vi "Tester.vi"(8 "error in (no error)":errorcluster, 11 "Selector in":refnum<class "Selector.lvclass">) -> (0 "error out":errorcluster, 3 "Selector out":refnum<class "Selector.lvclass">)   [LabVIEW 2019, in "Selector.lvclass"]
uses:
  Selector.lvclass
  <vilib>/Utility/miscctls.llb/LVPositionTypeDef.ctl
panel:
  out "Events":string[](array[string])
  in  "Multicolumn Listbox":i32(listbox)
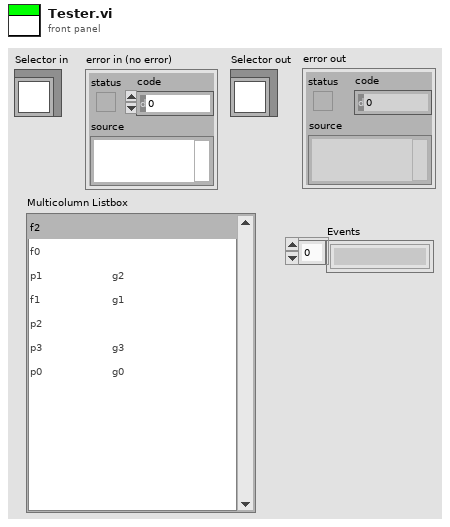
[diagram p1: front panel]
types:
  T1 = typedef "LVPositionTypeDef.ctl" = cluster{"Left":i32, "Top":i32}
  T2 = cluster{"Point":T1, "Button":u16, "PlatMods":cluster{"Shift":bool, "Ctrl":bool, "Alt":bool, "Cmd":bool, "Opt":bool}}
  T3 = enum32{"Invalid", "Standard", "Closed", "Hidden", "Minimized", "Maximized"}
  T4 = enum32{"invalid app kind", "Development System", "Run Time System", "Student Edition", "Embedded LabVIEW", "Evaluation", "Custom"}
  T5 = cluster{"Core":cluster{"Current VI Reference":refnum<vi>, "Close Panel on Exit?":bool}, "menu path":string}
  T6 = typedef "LVPoint32TypeDef.ctl" = cluster{"Horizontal":i32, "Vertical":i32}
  T7 = cluster{"Shift":bool, "Ctrl":bool, "Alt":bool, "Cmd":bool, "Opt":bool}
  T8 = cluster{"Current VI Reference":refnum<vi>, "Close Panel on Exit?":bool}
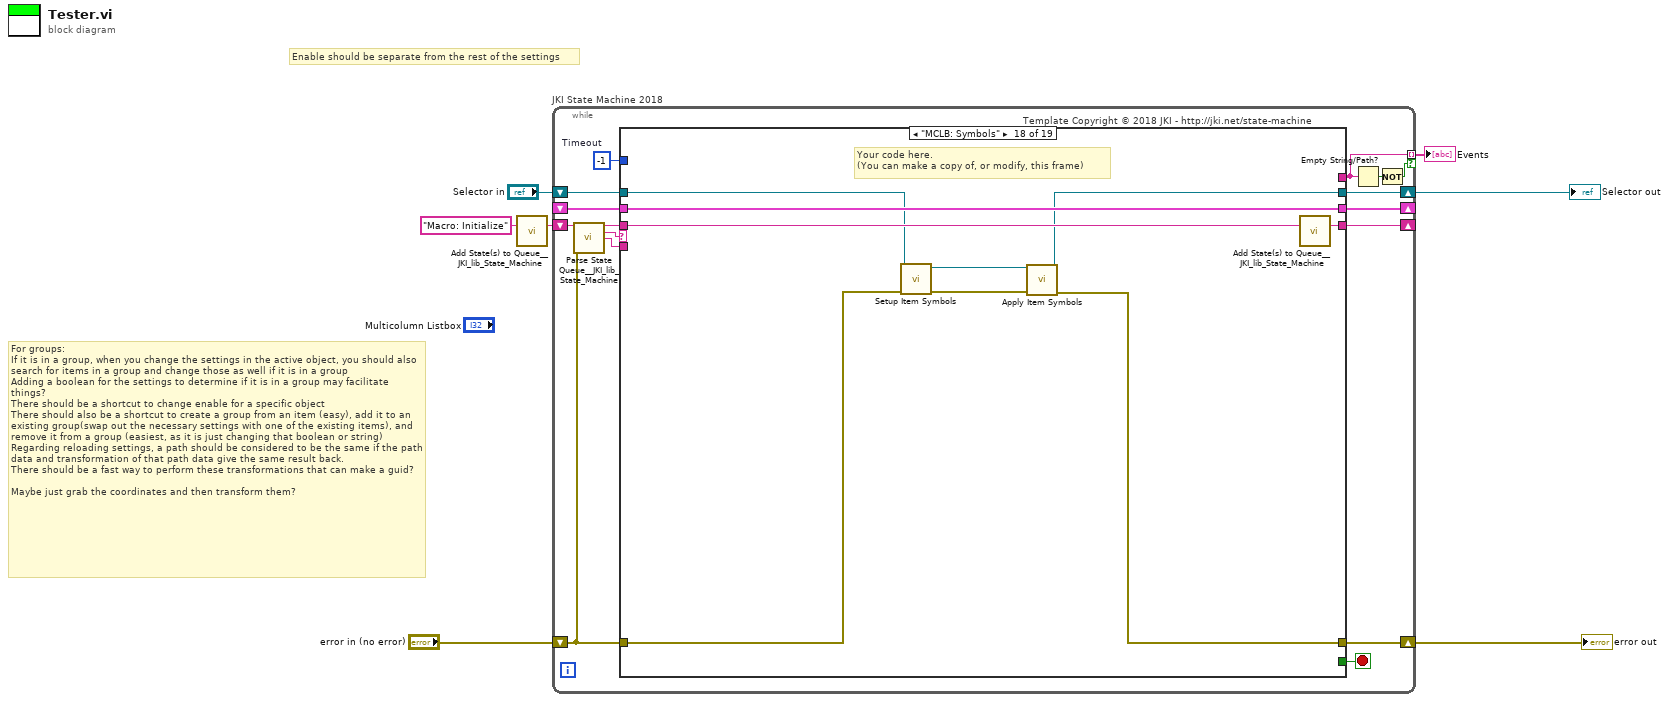
[diagram p0: block diagram]
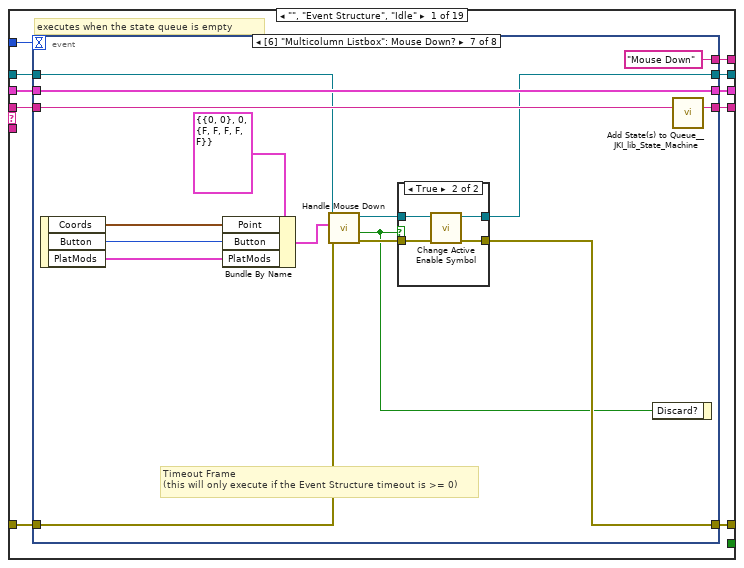
[diagram p2: hidden frame]
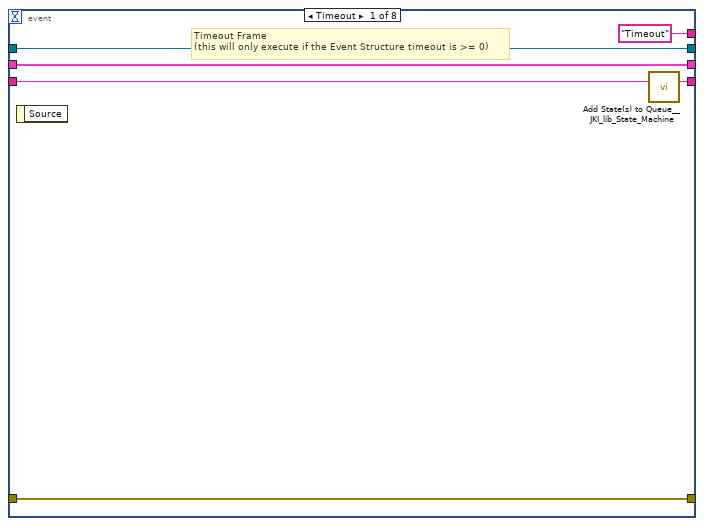
[diagram p3: hidden frame]
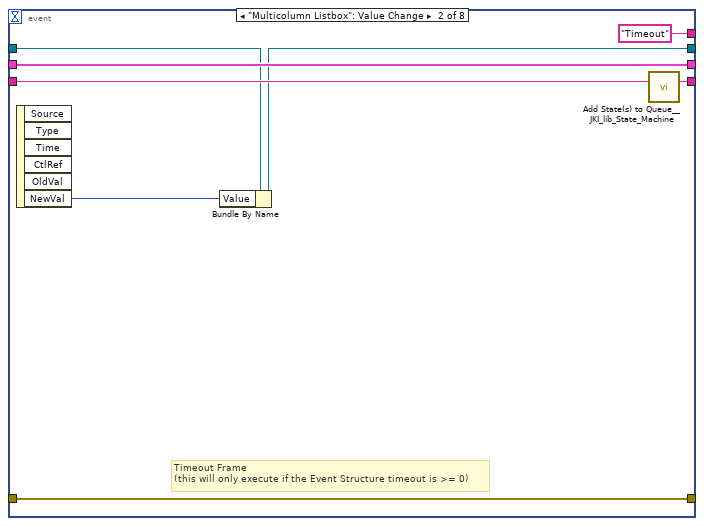
[diagram p4: hidden frame]
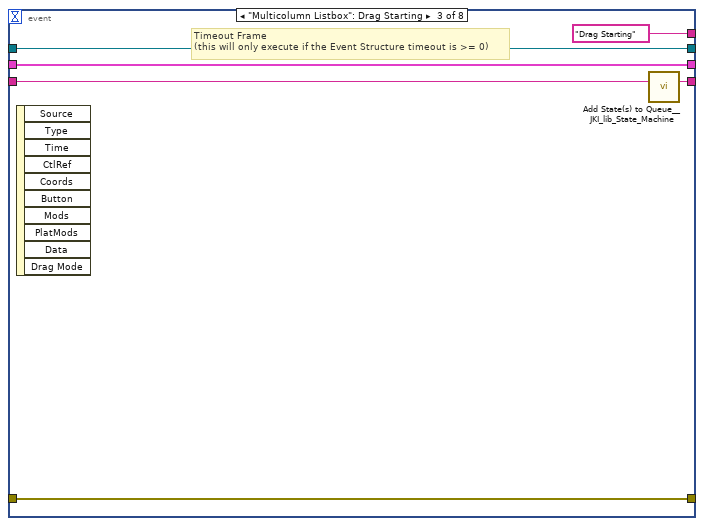
[diagram p5: hidden frame]
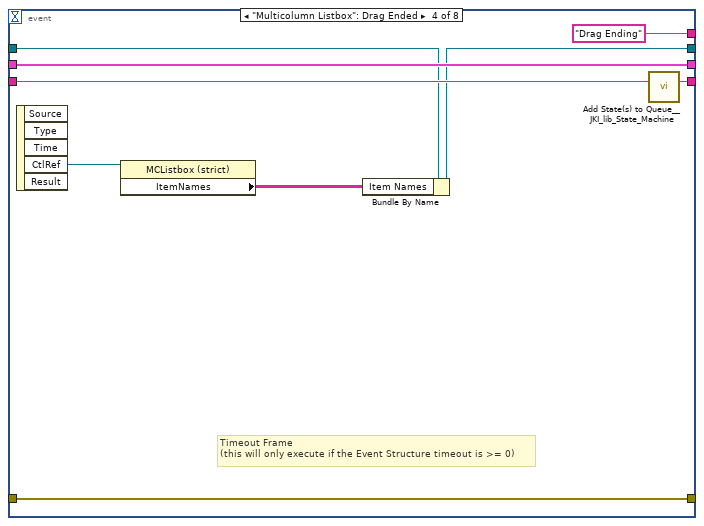
[diagram p6: hidden frame]
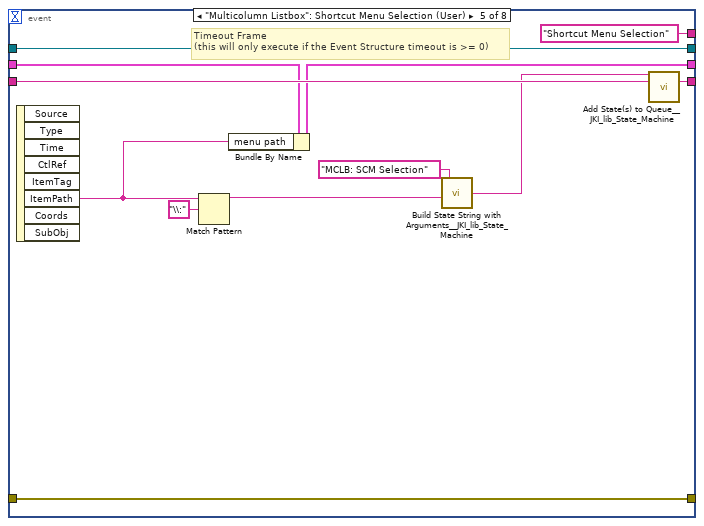
[diagram p7: hidden frame]
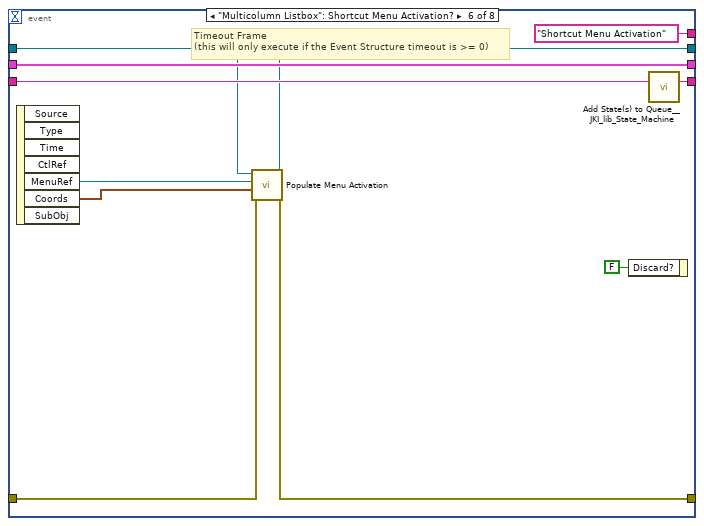
[diagram p8: hidden frame]
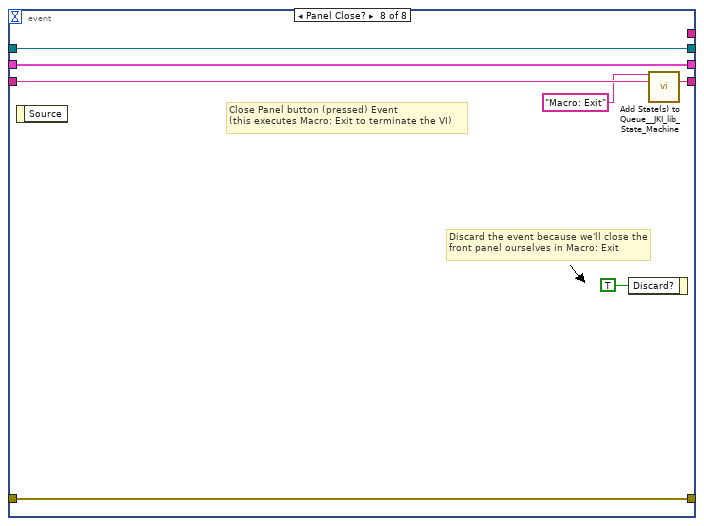
[diagram p10: hidden frame]
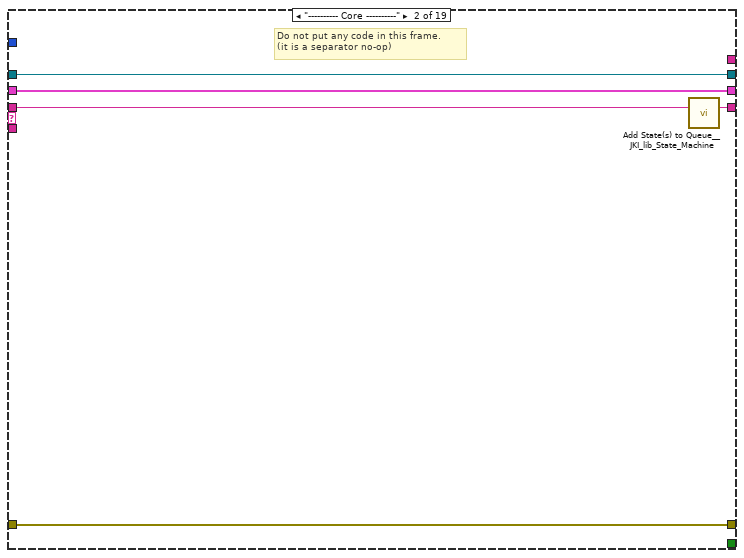
[diagram p11: hidden frame]
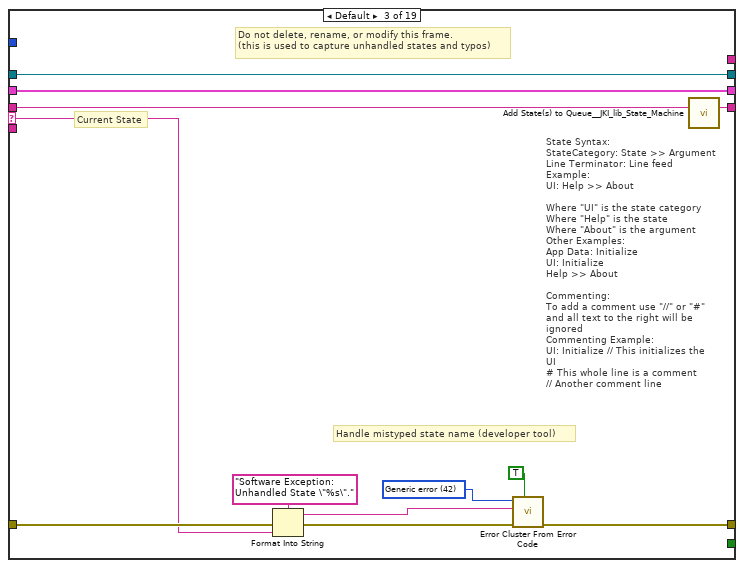
[diagram p12: hidden frame]
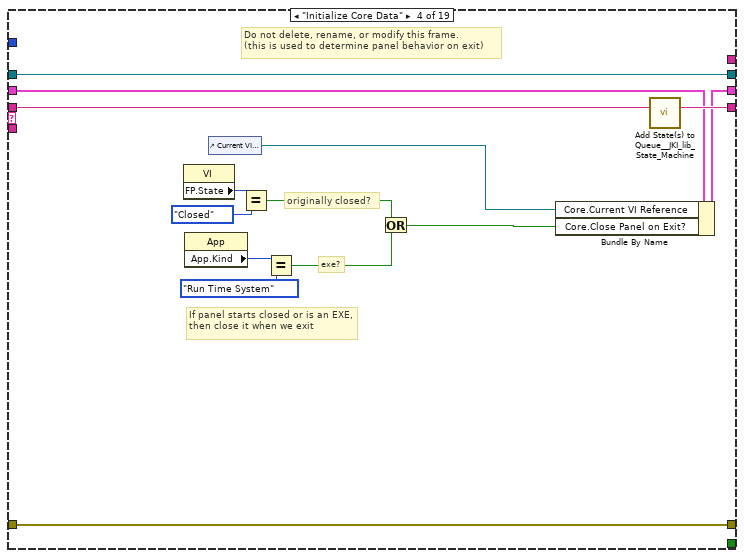
[diagram p13: hidden frame]
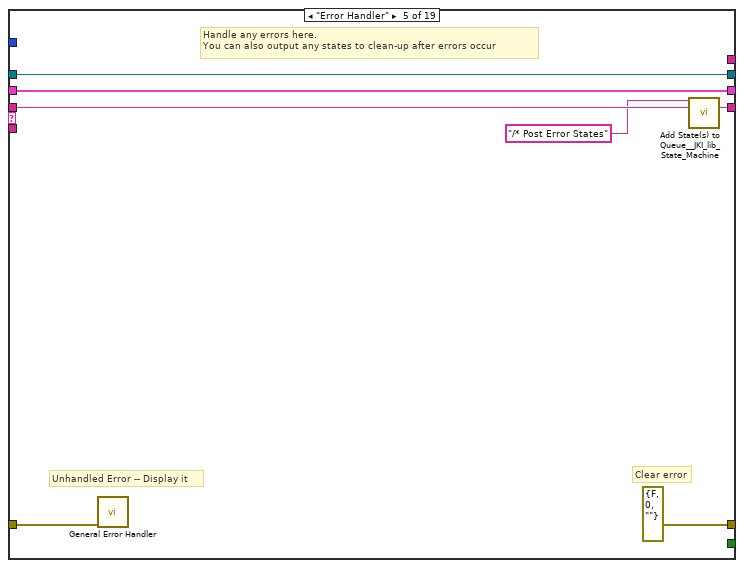
[diagram p14: hidden frame]
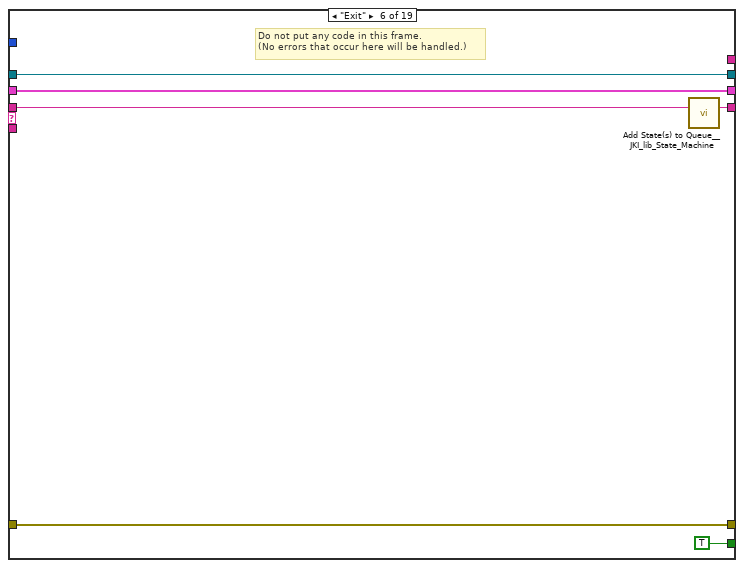
[diagram p15: hidden frame]
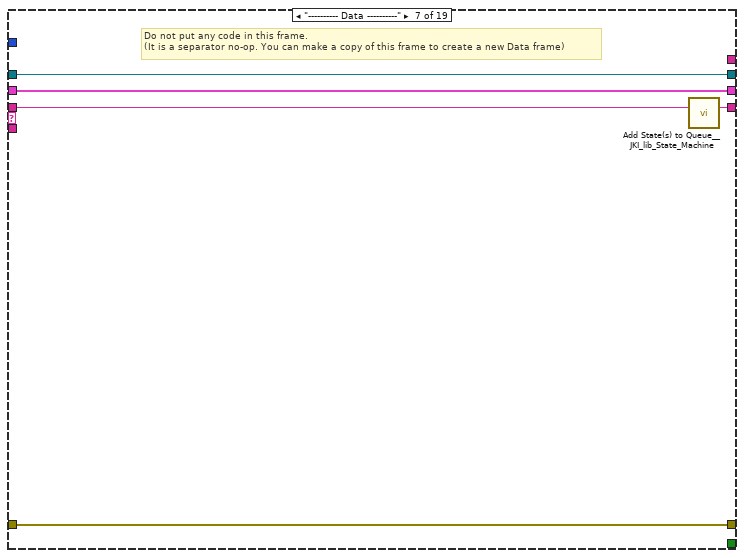
[diagram p16: hidden frame]
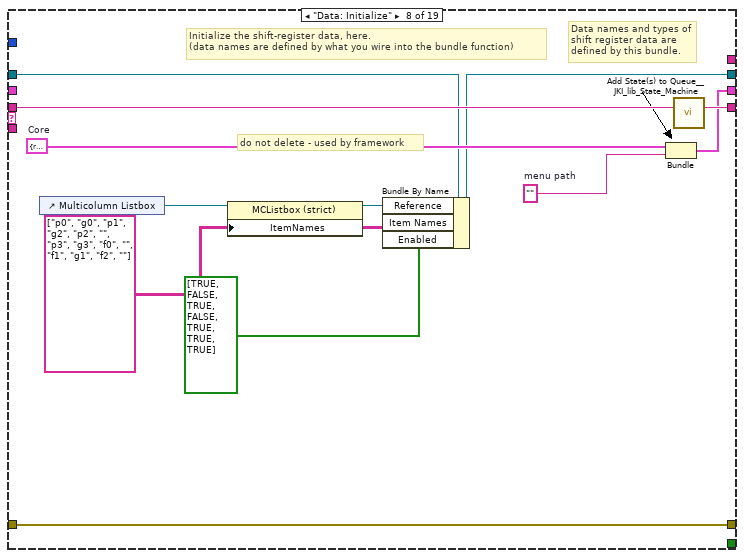
[diagram p17: hidden frame]
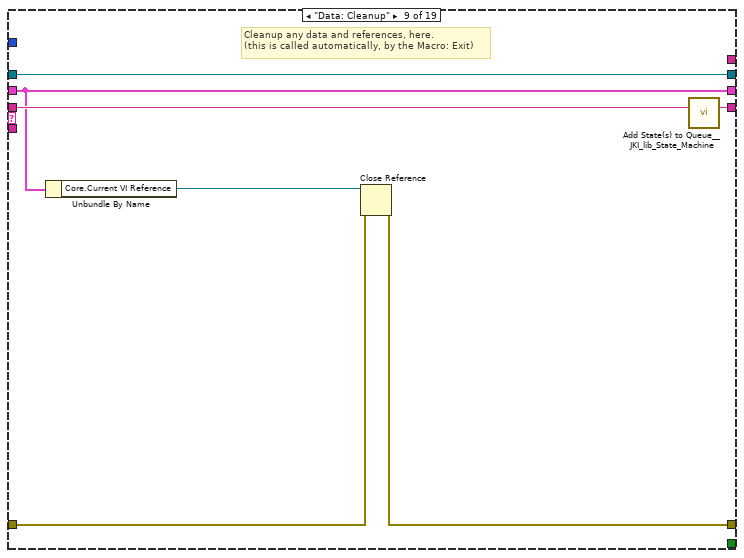
[diagram p18: hidden frame]
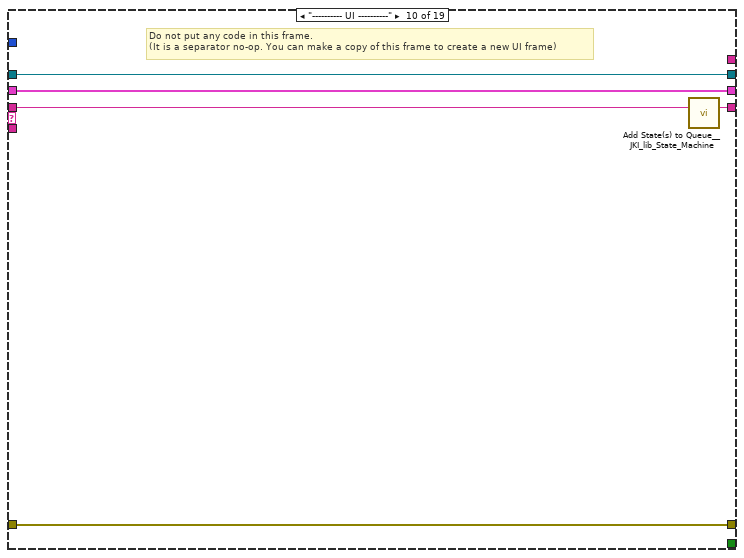
[diagram p19: hidden frame]
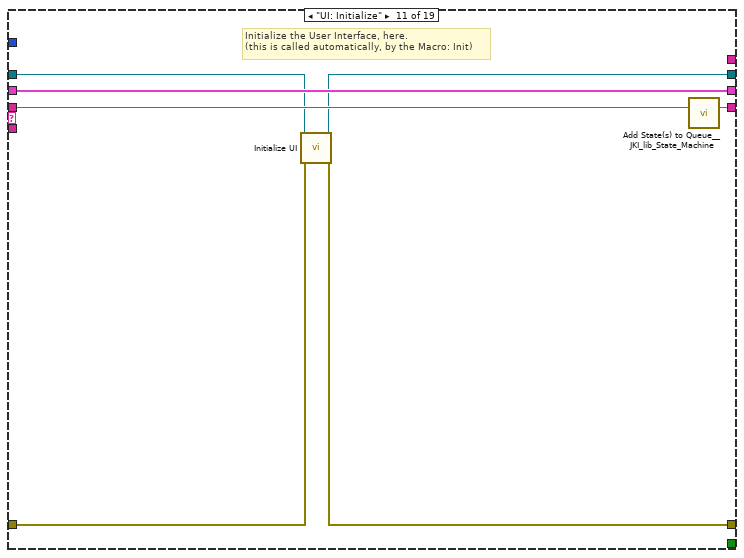
[diagram p20: hidden frame]
diagram:
  # "For groups:\nIf it is in a group, when you change the settings in the active object, you should also search for items in a group and change those as well if it is in a group \nAdding a boolean for the settings to determine if it is in a group may facilitate things?\nThere should be a shortcut to change enable for a specific object\nThere should also be a shortcut to create a group from an item (easy), add it to an existing group(swap out the necessary settings with one of the existing items), and remove it from a group (easiest, as it is just changing that boolean or string)\nRegarding reloading settings, a path should be considered to be the same if the path data and transformation of that path data give the same result back.\nThere should be a fast way to perform these transformations that can make a guid?\n\nMaybe just grab the coordinates and then transform them?"
  # "Enable should be separate from the rest of the settings"
  n1 = call <vilib>:"Add State(s) to Queue__JKI_lib_State_Machine.vi"("State(s) in (\"\")"="Macro: Initialize") -> ("States Out"=w7:string)  [unwired: 14 in]
  n2 = while "JKI State Machine 2018" {
    shift-right: [w16] -> _
    shift-left: _ -> [w15]
    shift-right: [w19] -> w2
    shift-left: "error in (no error)" -> [w13]
    shift-right: [w18] -> _
    shift-left: w7 -> [w20]
    shift-right: [w11] -> w4
    shift-left: "Selector in" -> [w12]
    tunnel: [w10] -> w1 mode=indexing if=w8
    stop <- w17 stop-if-true
    w14 = -1  # Timeout
    # "Template Copyright © 2018 JKI - http://jki.net/state-machine"
    n3 = call <vilib>:"Parse State Queue__JKI_lib_State_Machine.vi"("State Queue"=w20, "Error In (no error)"=w13) -> ("Remaining States"=w22:string, "Current State"=w23:string, "Arguments"=w21:string)  [unwired: 11 in]
    n4 = case shown="\"MCLB: Symbols\"" w23 {
      selector: w23 -> [_ _ w121 _ _ _ _ _ _ _ _ _ _ _ _ _ _ _ _]
      tunnel: w22 -> [w33 w119 w125 w145 w152 w158 w163 w175 w182 w187 w194 w201 w213 w283 w289 w300 w305 w314 w322]
      tunnel: w21 -> [_ _ _ _ _ _ _ _ _ _ _ w196 w207 _ _ _ _ _ w319]
      tunnel: w15 -> [w31 w116 w123 w138 w149 w156 w160 _ w177 w184 w192 w199 w209 w280 w286 w297 w302 w312 w316]
      tunnel: [w30 w117 w127 w142 errorcluster {"status"=FALSE, "code"=0, "source"=""} ("error out") w155 w161 w172 w178 w185 w189 w197 w210 w281 w287 w298 w303 w307 w320] -> w19
      tunnel: w13 -> [w29 w117 w126 w142 w148 w155 w161 w172 w179 w185 w188 w198 w211 w281 w287 w298 w303 w306 w320]
      tunnel: [w32 w118 w124 w144 w151 w157 w162 w174 w181 w186 w193 w200 w212 w282 w288 w299 w304 w313 w321] -> w18
      tunnel: [_ _ _ _ _ TRUE _ _ _ _ _ _ _ _ _ _ _ _ _] -> w17
      tunnel: [w28 w116 w123 w143 w149 w156 w160 w173 w177 w184 w192 w199 w209 w280 w286 w297 w302 w312 w316] -> w16
      tunnel: w14 -> [w27 _ _ _ _ _ _ _ _ _ _ _ _ _ _ _ _ _ _]
      tunnel: w12 -> [w26 w115 w120 w132 w146 w153 w159 w169 w176 w183 w190 w195 w206 w279 w284 w290 w301 w311 w317]
      tunnel: [w25 w115 w120 w132 w146 w153 w159 w170 w176 w183 w191 w195 w206 w279 w284 w290 w301 w308 w318] -> w11
      tunnel: [w24 _ _ _ _ _ _ _ _ _ _ _ _ _ _ _ _ _ _] -> w10
      frame "", "Event Structure", "Idle" {
        # "executes when the state queue is empty"
        n5 = event shown="[6] \"Multicolumn Listbox\": Mouse Down?" {
          selector: _ -> [_ _ _ _ _ _ _ _]
          dyn-events: _ -> [_ _ _ _ _ _ _ _]
          timeout: w27 -> [_ _ _ _ _ _ _ _]
          tunnel: w33 -> [w39 w47 w53 w62 w74 w85 w101 w114]
          tunnel: [w38 w46 w52 w61 w73 w84 w100 w113] -> w32
          tunnel: w31 -> [w36 w44 w50 w59 w67 w83 w99 w111]
          tunnel: [w37 w45 w51 w60 w72 w78 w91 w112] -> w30
          tunnel: w29 -> [w37 w45 w51 w60 w72 w77 w97 w112]
          tunnel: [w36 w44 w50 w59 w68 w83 w99 w111] -> w28
          tunnel: w26 -> [w35 w41 w49 w55 w71 w76 w98 w108]
          tunnel: [w35 w42 w49 w56 w71 w82 w89 w108] -> w25
          tunnel: ["Timeout" "Timeout" "Drag Starting" "Drag Ending" "Shortcut Menu Selection" "Shortcut Menu Activation" "Mouse Down" _] -> w24
          event Timeout {
            # "Timeout Frame\n(this will only execute if the Event Structure timeout is >= 0)"
            n6 = event-data() -> ()  [unwired: 1 in, 1 out]
            n7 = call <vilib>:"Add State(s) to Queue__JKI_lib_State_Machine.vi"("State(s) in (\"\")"=w39) -> ("States Out"=w38:string)  [unwired: 14 in]
          }
          event "Multicolumn Listbox": Value Change {
            # "Timeout Frame\n(this will only execute if the Event Structure timeout is >= 0)"
            n8 = event-data() -> ("NewVal"=w40:i32)  [unwired: 1 in, 5 out]
            n9 = Bundle By Name(cluster=w41, "Value"=w40) -> (w42:refnum<class "Selector.lvclass">)
            n10 = call <vilib>:"Add State(s) to Queue__JKI_lib_State_Machine.vi"("State(s) in (\"\")"=w47) -> ("States Out"=w46:string)  [unwired: 14 in]
          }
          event "Multicolumn Listbox": Drag Starting {
            # "Timeout Frame\n(this will only execute if the Event Structure timeout is >= 0)"
            n11 = event-data() -> ()  [unwired: 1 in, 10 out]
            n12 = call <vilib>:"Add State(s) to Queue__JKI_lib_State_Machine.vi"("State(s) in (\"\")"=w53) -> ("States Out"=w52:string)  [unwired: 14 in]
          }
          event "Multicolumn Listbox": Drag Ended {
            # "Timeout Frame\n(this will only execute if the Event Structure timeout is >= 0)"
            n13 = event-data() -> ("CtlRef"=w57:refnum<vi>)  [unwired: 1 in, 4 out]
            n14 = property class="MCListbox (strict)"(reference=w57) -> ("ItemNames"=w54:string[][])  [unwired: 1 in, 2 out]
            n15 = Bundle By Name(cluster=w55, "Item Names"=w54) -> (w56:refnum<class "Selector.lvclass">)
            n16 = call <vilib>:"Add State(s) to Queue__JKI_lib_State_Machine.vi"("State(s) in (\"\")"=w62) -> ("States Out"=w61:string)  [unwired: 14 in]
          }
          event "Multicolumn Listbox": Shortcut Menu Selection (User) {
            # "Timeout Frame\n(this will only execute if the Event Structure timeout is >= 0)"
            n17 = event-data() -> ("ItemPath"=w69:string)  [unwired: 1 in, 7 out]
            n18 = Match Pattern(string=w69, regular expression="\\:") -> (before substring=w65:string)  [unwired: 1 in, 3 out]
            n19 = Bundle By Name(cluster=w67, "menu path"=w69) -> (w68:T5)
            n20 = call <vilib>:"Build State String with Arguments__JKI_lib_State_Machine.vi"("Arguments (\"\")"=w65, "State"="MCLB: SCM Selection") -> ("State with Arguments"=w64:string)  [unwired: 4 in]
            n21 = call <vilib>:"Add State(s) to Queue__JKI_lib_State_Machine.vi"("State(s) in Front (\"\")"=w64, "State(s) in (\"\")"=w74) -> ("States Out"=w73:string)  [unwired: 13 in]
          }
          event "Multicolumn Listbox": Shortcut Menu Activation? {
            # "Timeout Frame\n(this will only execute if the Event Structure timeout is >= 0)"
            n22 = event-data() -> ("MenuRef"=w81:refnum<k9>, "Coords"=w80:T6)  [unwired: 1 in, 5 out]
            n23 = call-dynamic "Populate Menu Activation.vi"("error in (no error)"=w77, "Point32"=w80, "MenuRef"=w81, "Selector in"=w76) -> ("error out"=w78:errorcluster, "Selector out"=w82:refnum<class "Selector.lvclass">)  [unwired: 6 in]
            n24 = event-data("Discard?"=FALSE) -> ()  [unwired: 1 in, 1 out]
            n25 = call <vilib>:"Add State(s) to Queue__JKI_lib_State_Machine.vi"("State(s) in (\"\")"=w85) -> ("States Out"=w84:string)  [unwired: 14 in]
          }
          event "Multicolumn Listbox": Mouse Down? {
            # "Timeout Frame\n(this will only execute if the Event Structure timeout is >= 0)"
            n26 = event-data() -> ("Coords"=w94:T6, "Button"=w93:u16, "PlatMods"=w95:T7)  [unwired: 1 in]
            n27 = Bundle By Name(cluster=T2 {"Point"={"Left"=0, "Top"=0}, "Button"=0, "PlatMods"={"Shift"=FALSE, "Ctrl"=FALSE, "Alt"=FALSE, "Cmd"=FALSE, "Opt"=FALSE}} ("Event Data"), "Point"=w94, "Button"=w93, "PlatMods"=w95) -> (w86:T2)
            n28 = call-dynamic "Handle Mouse Down.vi"("error in (no error)"=w97, "Event Data"=w86, "Selector in"=w98) -> ("error out"=w92:errorcluster, "Enable Change"=w87:bool, "Selector out"=w90:refnum<class "Selector.lvclass">)  [unwired: 6 in]
            n29 = case shown="True" w87 {
              tunnel: w90 -> [w103 w107]
              tunnel: w92 -> [w102 w106]
              tunnel: [w102 w105] -> w91
              tunnel: [w103 w104] -> w89
              frame False {
              }
              frame True {
                n30 = call "Change Active Enable Symbol.vi"("error in (no error)"=w106, "Selector in"=w107) -> ("error out"=w105:errorcluster, "Selector out"=w104:refnum<class "Selector.lvclass">)  [unwired: 8 in]
              }
            }
            n31 = event-data("Discard?"=w87) -> ()  [unwired: 1 in, 1 out]
            n32 = call <vilib>:"Add State(s) to Queue__JKI_lib_State_Machine.vi"("State(s) in (\"\")"=w101) -> ("States Out"=w100:string)  [unwired: 14 in]
          }
          event Panel Close? {
            # "Discard the event because we'll close the front panel ourselves in Macro: Exit"
            # "Close Panel button (pressed) Event\n(this executes Macro: Exit to terminate the VI)"
            n33 = event-data() -> ()  [unwired: 1 in, 1 out]
            n34 = event-data("Discard?"=TRUE) -> ()  [unwired: 1 in, 1 out]
            n35 = call <vilib>:"Add State(s) to Queue__JKI_lib_State_Machine.vi"("State(s) in Front (\"\")"="Macro: Exit", "State(s) in (\"\")"=w114) -> ("States Out"=w113:string)  [unwired: 13 in]
          }
        }
      }
      frame "---------- Core ----------" {
        # "Do not put any code in this frame.\n(it is a separator no-op)"
        n36 = call <vilib>:"Add State(s) to Queue__JKI_lib_State_Machine.vi"("State(s) in (\"\")"=w119) -> ("States Out"=w118:string)  [unwired: 14 in]
      }
      frame Default {
        w130 = 42 items=["No error", "Argument error", "Memory is full", "Out of zone", "End of file", "File already open", "Generic file I/O error", "File not found", "File permission error", "Disk is full", "Duplicate path", "Too many files open", "System feature not enabled", "Resource file not found", "Cannot add resource", "Resource not found", "Image not found", "Image memory error", "Pen does not exist", "Config type invalid", "Config token not found", "Config parse error", "Config memory error", "Bad external code format", "Bad external code offset", "External code not present", "Null window", "Destroy window error", "Null menu", "Print aborted", "Bad print record", "Print driver error", "Windows error during printing", "Memory error during printing", "Print dialog error", "Generic print error", "Invalid device refnum", "Device not found", "Device parameter error", "Device unit error", "Cannot open device", "Device call aborted", "Generic error", "Cancelled by user", "Object ID too low", "Object ID too high", "Object not in heap", "Unknown heap", "Unknown object (invalid DefProc)", "Unknown object (DefProc not in table)", "Message out of range", "Invalid (null) method", "Unknown message", "Manager call not supported", "Bad address", "Network operation in progress", "Network operation timed out", "Connection is busy", "Network attribute not supported", "Network error", "Address in use", "System out of memory", "Connection aborted", "Connection refused", "Not connected", "Already connected", "Connection closed", "Initialization error (interapplication manager)", "Bad occurrence", "Wait on unbound occurrence handler", "Occurrence queue overflow", "Datalog type conflict", "Unused", "Unrecognized type (interapplication manager)", "Memory corrupt", "Failed to make temporary DLL", "Old CIN version", "Drag socket not found", "Failed to load drop-object", "Failed to register OLE object", "Failed to release OLE object", "Format specifier type mismatch", "Unknown format specifier", "Too few format specifiers", "Too many format specifiers", "Scan failed", "Newer CIN version", "Error converting to variant", "Runtime menu error", "Password tampered", "Variant attribute not found", "Incompatible variant data type", "Event data is not available", "Event Store is not present", "Occurrence is not found", "Event Queue is not created", "Event info is not available", "Refnum passed is NULL", "Error retrieving Class GUID", "Error retrieving CoClass GUID", "Error retrieving TypeLib GUID.", "Bad built application magic bytes.", "Specific driver is different from the specific driver associated with the Logical Name.", "There is no session opened to the class driver.", "Max Error", "MAX - Error with config objects", "MAX - Error loading configuration", "MAX - Group not supported"]
        # "State Syntax:\nStateCategory: State >> Argument\nLine Terminator: Line feed\nExample:\nUI: Help >> About\n\nWhere \"UI\" is the state category\nWhere \"Help\" is the state\nWhere \"About\" is the argument\nOther Examples:\nApp Data: Initialize\nUI: Initialize\nHelp >> About\n\nCommenting:\nTo add a comment use \"//\" or \"#\" and all text to the right will be ignored\nCommenting Example:\nUI: Initialize // This initializes the UI\n# This whole line is a comment\n// Another comment line"
        # "Current State"
        # "Do not delete, rename, or modify this frame.\n(this is used to capture unhandled states and typos)"
        # "Handle mistyped state name (developer tool)"
        n37 = Format Into String(format string="Software Exception: Unhandled State \"%s\"." ("message"), error in=w126, w121) -> (resulting string=w129:string, error out=w128:errorcluster)  [unwired: 1 in]
        n38 = call <vilib>:"Error Cluster From Error Code.vi"("show call chain? (False)"=TRUE, "error in (no error)"=w128, "error message (\"\")"=w129, "error code (0)"=w130) -> ("error out"=w127:errorcluster)  [unwired: 5 in]
        n39 = call <vilib>:"Add State(s) to Queue__JKI_lib_State_Machine.vi"("State(s) in (\"\")"=w125) -> ("States Out"=w124:string)  [unwired: 14 in]
      }
      frame "Initialize Core Data" {
        # "Do not delete, rename, or modify this frame.\n(this is used to determine panel behavior on exit)"
        # "originally closed?"
        # "exe?"
        # "If panel starts closed or is an EXE, then close it when we exit"
        n40 = property class="VI"() -> ("FP.State"=w135:T3)  [unwired: 2 in, 2 out]
        n41 = property class="App"() -> ("App.Kind"=w141:T4)  [unwired: 2 in, 2 out]
        n42 = control-ref of="Current VI Reference"() -> (w136:refnum<vi>)
        n43 = Equal?(x=w135, y=T3."Closed" ("Front Panel Window:State")) -> (x = y?=w133:bool)
        n44 = Equal?(x=w141, y=T4."Run Time System" ("Application:Kind")) -> (x = y?=w139:bool)
        n45 = Or(x=w133, y=w139) -> (x .or. y?=w137:bool)
        n46 = Bundle By Name(cluster=w138, "Core.Current VI Reference"=w136, "Core.Close Panel on Exit?"=w137) -> (w143:T5)
        n47 = call <vilib>:"Add State(s) to Queue__JKI_lib_State_Machine.vi"("State(s) in (\"\")"=w145) -> ("States Out"=w144:string)  [unwired: 14 in]
      }
      frame "Error Handler" {
        # "Unhandled Error -- Display it"
        # "Handle any errors here.\nYou can also output any states to clean-up after errors occur"
        # "Clear error"
        n48 = call <vilib>:"General Error Handler.vi"("error in (no error)"=w148) -> ()  [unwired: 10 in, 5 out]
        n49 = call <vilib>:"Add State(s) to Queue__JKI_lib_State_Machine.vi"("State(s) in Front (\"\")"="/* Post Error States", "State(s) in (\"\")"=w152) -> ("States Out"=w151:string)  [unwired: 13 in]
      }
      frame "Exit" {
        # "Do not put any code in this frame.\n(No errors that occur here will be handled.)"
        n50 = call <vilib>:"Add State(s) to Queue__JKI_lib_State_Machine.vi"("State(s) in (\"\")"=w158) -> ("States Out"=w157:string)  [unwired: 14 in]
      }
      frame "---------- Data ----------" {
        # "Do not put any code in this frame.\n(It is a separator no-op. You can make a copy of this frame to create a new Data frame)"
        n51 = call <vilib>:"Add State(s) to Queue__JKI_lib_State_Machine.vi"("State(s) in (\"\")"=w163) -> ("States Out"=w162:string)  [unwired: 14 in]
      }
      frame "Data: Initialize" {
        w164 = ""  # menu path
        w166 = string[][] [["p0", "g0"], ["p1", "g2"], ["p2", ""], ["p3", "g3"], ["f0", ""], ["f1", "g1"], ["f2", ""]] ("Item Names")
        w171 = T8 {"Current VI Reference"=refnum, "Close Panel on Exit?"=FALSE}  # Core
        # "do not delete - used by framework"
        # "Data names and types of shift register data are defined by this bundle."
        # "Initialize the shift-register data, here.\n(data names are defined by what you wire into the bundle function)"
        n52 = control-ref of="Multicolumn Listbox"() -> (w168:refnum<vi>)
        n53 = property class="MCListbox (strict)"(reference=w168, "ItemNames"=w166) -> (reference out=w167:refnum<vi>)  [unwired: 1 in, 1 out]
        n54 = Bundle By Name(cluster=w169, "Reference"=w167, "Item Names"=w166, "Enabled"=bool[] [TRUE, FALSE, TRUE, FALSE, TRUE, TRUE, TRUE]) -> (w170:refnum<class "Selector.lvclass">)
        n55 = Bundle("Core"=w171, "menu path"=w164) -> (w173:T5)  [unwired: 1 in]
        n56 = call <vilib>:"Add State(s) to Queue__JKI_lib_State_Machine.vi"("State(s) in (\"\")"=w175) -> ("States Out"=w174:string)  [unwired: 14 in]
      }
      frame "Data: Cleanup" {
        # "Cleanup any data and references, here.\n(this is called automatically, by the Macro: Exit)"
        n57 = Unbundle By Name(w177) -> ("Core.Current VI Reference"=w180:refnum<vi>)
        n58 = Close Reference(reference=w180, error in (no error)=w179) -> (error out=w178:errorcluster)
        n59 = call <vilib>:"Add State(s) to Queue__JKI_lib_State_Machine.vi"("State(s) in (\"\")"=w182) -> ("States Out"=w181:string)  [unwired: 14 in]
      }
      frame "---------- UI ----------" {
        # "Do not put any code in this frame.\n(It is a separator no-op. You can make a copy of this frame to create a new UI frame)"
        n60 = call <vilib>:"Add State(s) to Queue__JKI_lib_State_Machine.vi"("State(s) in (\"\")"=w187) -> ("States Out"=w186:string)  [unwired: 14 in]
      }
      frame "UI: Initialize" {
        # "Initialize the User Interface, here.\n(this is called automatically, by the Macro: Init)"
        n61 = call-dynamic "Initialize UI.vi"("error in (no error)"=w188, "Selector in"=w190) -> ("error out"=w189:errorcluster, "Selector out"=w191:refnum<class "Selector.lvclass">)  [unwired: 8 in]
        n62 = call <vilib>:"Add State(s) to Queue__JKI_lib_State_Machine.vi"("State(s) in (\"\")"=w194) -> ("States Out"=w193:string)  [unwired: 14 in]
      }
      frame "UI: Cursor Set" {
        # "Argument"
        # "Set and Unset Cursor Busy.\n(Usage: \"UI: Cursor Set >> Busy|Idle\")"
        n63 = case shown="\"Idle\", Default" w196 {
          tunnel: w198 -> [w203 w205]
          tunnel: [w202 w204] -> w197
          frame "Idle", Default {
            n64 = call <vilib>:"Unset Busy.vi"("error in (no error)"=w203) -> ("error out"=w202:errorcluster)  [unwired: 10 in]
          }
          frame "Busy" {
            n65 = call <vilib>:"Set Busy.vi"("error in (no error)"=w205) -> ("error out"=w204:errorcluster)  [unwired: 9 in, 1 out]
          }
        }
        n66 = call <vilib>:"Add State(s) to Queue__JKI_lib_State_Machine.vi"("State(s) in (\"\")"=w201) -> ("States Out"=w200:string)  [unwired: 14 in]
      }
      frame "UI: Front Panel State" {
        # "Argument"
        # "Set Front Panel Open or Closed\n(Usage: \"UI: Front Panel State >> Open|Close\")"
        n67 = Unbundle By Name(w209) -> ("Core.Current VI Reference"=w208:refnum<vi>)
        n68 = case shown="\"Minimize\", \"Minimized\"" w207 {
          tunnel: w211 -> [w219 w234 w245 w258 w271]
          tunnel: [w221 w235 w247 w260 w273] -> w210
          tunnel: w208 -> [w220 w232 w246 w259 w272]
          frame "Open", "Standard", Default {
            w214 = T3."Standard" ("State")
            n69 = property class="VI"(reference=w220, error in=w219) -> (reference out=w217:refnum<vi>, error out=w218:errorcluster, "FP.State"=w216:T3)
            n70 = Not Equal?(x=w216, y=w214) -> (x != y?=w215:bool)
            n71 = case shown="True" w215 {
              tunnel: [w225 w227] -> w221
              tunnel: w218 -> [w224 w227]
              tunnel: w217 -> [w223 _]
              tunnel: w214 -> [w222 _]
              frame True {
                n72 = invoke class="VI" method="FP.Open"(reference=w223, error in=w224, "Activate"=TRUE, "State"=w222) -> (error out=w225:errorcluster)  [unwired: 1 in, 4 out]
              }
              frame False {
              }
            }
          }
          frame "Close", "Closed" {
            n73 = property class="VI"(reference=w232, error in=w234) -> (reference out=w231:refnum<vi>, error out=w233:errorcluster, "FP.State"=w229:T3)
            n74 = Not Equal?(x=w229, y=T3."Closed" ("Front Panel Window:State")) -> (x != y?=w228:bool)
            n75 = case shown="True" w228 {
              tunnel: [w236 w239] -> w235
              tunnel: w233 -> [w236 w238]
              tunnel: w231 -> [_ w237]
              frame False {
              }
              frame True {
                n76 = invoke class="VI" method="FP.Close"(reference=w237, error in=w238) -> (error out=w239:errorcluster)  [unwired: 1 in, 2 out]
              }
            }
          }
          frame "Hidden", "Hide" {
            w240 = T3."Hidden" ("State")
            n77 = property class="VI"(reference=w246, error in=w245) -> (reference out=w243:refnum<vi>, error out=w244:errorcluster, "FP.State"=w242:T3)
            n78 = Not Equal?(x=w242, y=w240) -> (x != y?=w241:bool)
            n79 = case shown="True" w241 {
              tunnel: [w251 w252] -> w247
              tunnel: w244 -> [w250 w252]
              tunnel: w243 -> [w249 _]
              tunnel: w240 -> [w248 _]
              frame True {
                n80 = invoke class="VI" method="FP.Open"(reference=w249, error in=w250, "State"=w248) -> (error out=w251:errorcluster)  [unwired: 2 in, 4 out]
              }
              frame False {
              }
            }
          }
          frame "Minimize", "Minimized" {
            w253 = T3."Minimized" ("State")
            n81 = property class="VI"(reference=w259, error in=w258) -> (reference out=w256:refnum<vi>, error out=w257:errorcluster, "FP.State"=w255:T3)
            n82 = Not Equal?(x=w255, y=w253) -> (x != y?=w254:bool)
            n83 = case shown="True" w254 {
              tunnel: [w264 w265] -> w260
              tunnel: w257 -> [w263 w265]
              tunnel: w256 -> [w262 _]
              tunnel: w253 -> [w261 _]
              frame True {
                n84 = invoke class="VI" method="FP.Open"(reference=w262, error in=w263, "State"=w261) -> (error out=w264:errorcluster)  [unwired: 2 in, 4 out]
              }
              frame False {
              }
            }
          }
          frame "Maximize", "Maximized" {
            w266 = T3."Maximized" ("State")
            n85 = property class="VI"(reference=w272, error in=w271) -> (reference out=w269:refnum<vi>, error out=w270:errorcluster, "FP.State"=w268:T3)
            n86 = Not Equal?(x=w268, y=w266) -> (x != y?=w267:bool)
            n87 = case shown="True" w267 {
              tunnel: [w277 w278] -> w273
              tunnel: w270 -> [w276 w278]
              tunnel: w269 -> [w275 _]
              tunnel: w266 -> [w274 _]
              frame True {
                n88 = invoke class="VI" method="FP.Open"(reference=w275, error in=w276, "State"=w274) -> (error out=w277:errorcluster)  [unwired: 2 in, 4 out]
              }
              frame False {
              }
            }
          }
        }
        n89 = call <vilib>:"Add State(s) to Queue__JKI_lib_State_Machine.vi"("State(s) in (\"\")"=w213) -> ("States Out"=w212:string)  [unwired: 14 in]
      }
      frame "---------- Macro ----------" {
        # "Do not put any code in this frame.\n(It is a separator no-op. You can make a copy of this frame to create a new Macro frame)"
        n90 = call <vilib>:"Add State(s) to Queue__JKI_lib_State_Machine.vi"("State(s) in (\"\")"=w283) -> ("States Out"=w282:string)  [unwired: 14 in]
      }
      frame "Macro: Initialize" {
        # "Initialization Macro\n(This is called once, when the VI starts)"
        n91 = call <vilib>:"Add State(s) to Queue__JKI_lib_State_Machine.vi"("State(s) in Front (\"\")"="Data: Initialize\nInitialize Core Data\nUI: Initialize\nUI: Front Panel State >> Open\nMCLB: Symbols", "State(s) in (\"\")"=w289) -> ("States Out"=w288:string)  [unwired: 13 in]
      }
      frame "Macro: Exit" {
        # "Exit Macro\n(This is called once, when the VI exits)"
        n92 = Unbundle By Name(w297) -> ("Core.Close Panel on Exit?"=w296:bool)
        n93 = Select(t="UI: Front Panel State >> Close", s=w296, f="") -> (s? t:f=w293:string)
        n94 = call <vilib>:"Add State(s) to Queue__JKI_lib_State_Machine.vi"("State(s) in (\"\")"=w293, "State(s) at Back (\"\")"="Data: Cleanup\nExit") -> ("States Out"=w291:string)  [unwired: 13 in]
        n95 = call <vilib>:"Add State(s) to Queue__JKI_lib_State_Machine.vi"("State(s) in Front (\"\")"=w291, "State(s) in (\"\")"=w300) -> ("States Out"=w299:string)  [unwired: 13 in]
      }
      frame "---------- MCLB ----------" {
        # "Template Separator\n(You can make a copy of, or modify, this frame)"
        n96 = call <vilib>:"Add State(s) to Queue__JKI_lib_State_Machine.vi"("State(s) in (\"\")"=w305) -> ("States Out"=w304:string)  [unwired: 14 in]
      }
      frame "MCLB: Symbols" {
        # "Your code here.\n(You can make a copy of, or modify, this frame)"
        n97 = call-dynamic "Setup Item Symbols.vi"("error in (no error)"=w306, "Selector in"=w311) -> ("error out"=w310:errorcluster, "Selector out"=w309:refnum<class "Selector.lvclass">)  [unwired: 8 in]
        n98 = call-dynamic "Apply Item Symbols.vi"("error in (no error)"=w310, "Selector in"=w309) -> ("error out"=w307:errorcluster, "Selector out"=w308:refnum<class "Selector.lvclass">)  [unwired: 8 in]
        n99 = call <vilib>:"Add State(s) to Queue__JKI_lib_State_Machine.vi"("State(s) in (\"\")"=w314) -> ("States Out"=w313:string)  [unwired: 14 in]
      }
      frame "MCLB: SCM Selection" {
        # "Your code here.\n(You can make a copy of, or modify, this frame)"
        n100 = Unbundle By Name(w316) -> ("menu path"=w315:string)
        n101 = case shown="\"add\"" w319 {
          tunnel: w317 -> [w323 w325 w327 w330]
          tunnel: [w323 w326 w328 w329] -> w318
          tunnel: w315 -> [_ w324 _ _]
          frame Default {
          }
          frame "add" {
            n102 = call "Add Item to Group.vi"("Menu Path"=w324, "Selector in"=w325) -> ("Selector out"=w326:refnum<class "Selector.lvclass">)  [unwired: 8 in, 1 out]
          }
          frame "create" {
            n103 = call-dynamic "Create New Group.vi"("Selector in"=w327) -> ("Selector out"=w328:refnum<class "Selector.lvclass">)  [unwired: 9 in, 1 out]
          }
          frame "remove" {
            n104 = call-dynamic "Remove Item From Group.vi"("Selector in"=w330) -> ("Selector out"=w329:refnum<class "Selector.lvclass">)  [unwired: 9 in, 1 out]
          }
        }
        n105 = call <vilib>:"Add State(s) to Queue__JKI_lib_State_Machine.vi"("State(s) in (\"\")"=w322) -> ("States Out"=w321:string)  [unwired: 14 in]
      }
    }
    n106 = Empty String/Path?(string/path=w10) -> (empty?=w9:bool)
    n107 = Not(x=w9) -> (.not. x?=w8:bool)
  }
  "error out" <- w2
  "Selector out" <- w4
  "Events" <- w1
